vi "GEA3 HEWH Inverter ERD List.vi"(8 "error in (no error)":errorcluster, 11 "Enable Inverter ERD List":bool) -> (0 "error out":errorcluster, 2 "Headers":string[](array[string]), 3 "Read ERD List":T1[](array[typedef]) {"ERD Number" format="%.0x"})   [LabVIEW 2023]
uses:
  type defs/ERD Read Data In.ctl
  type defs/Data Type.ctl
  <vilib>/Utility/error.llb/whitespace.ctl
  <vilib>/Utility/error.llb/Trim Whitespace One-Sided.vi
  library/GEA2_Toolkit.lvlib
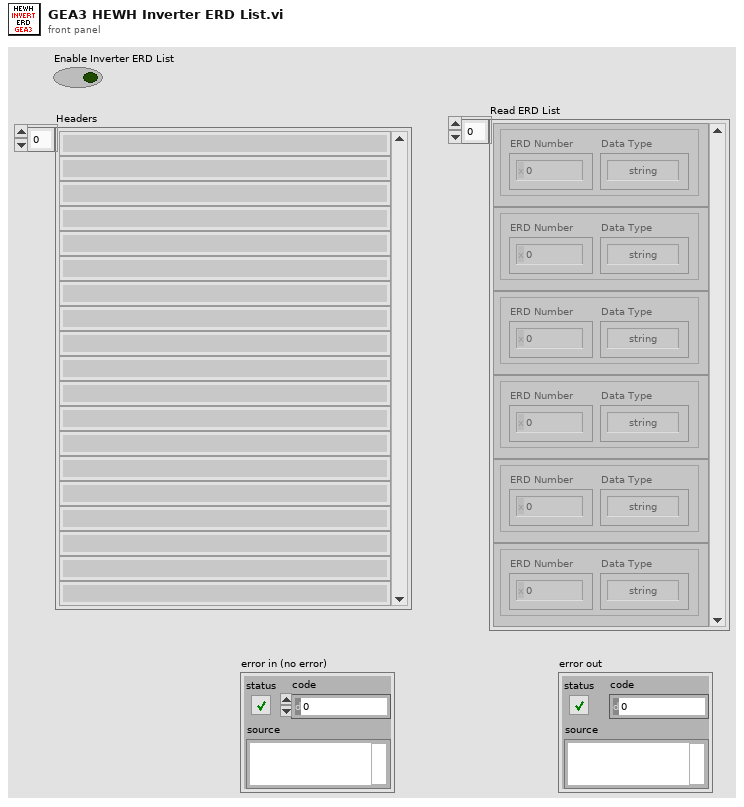
[diagram p1: front panel]
types:
  T1 = typedef "GEA2_Toolkit.lvlib/ERD Read Data In.ctl" = cluster{"ERD Number":u16, "Data Type":T2}
  T2 = typedef "GEA2_Toolkit.lvlib/Data Type.ctl" = enum16{"string", "boolean", "uint8_t", "uint16_t", "uint32_t", "uint64_t", "int8_t", "int16_t", "int32_t", "int64_t"}
  T3 = typedef "whitespace.ctl" = u16
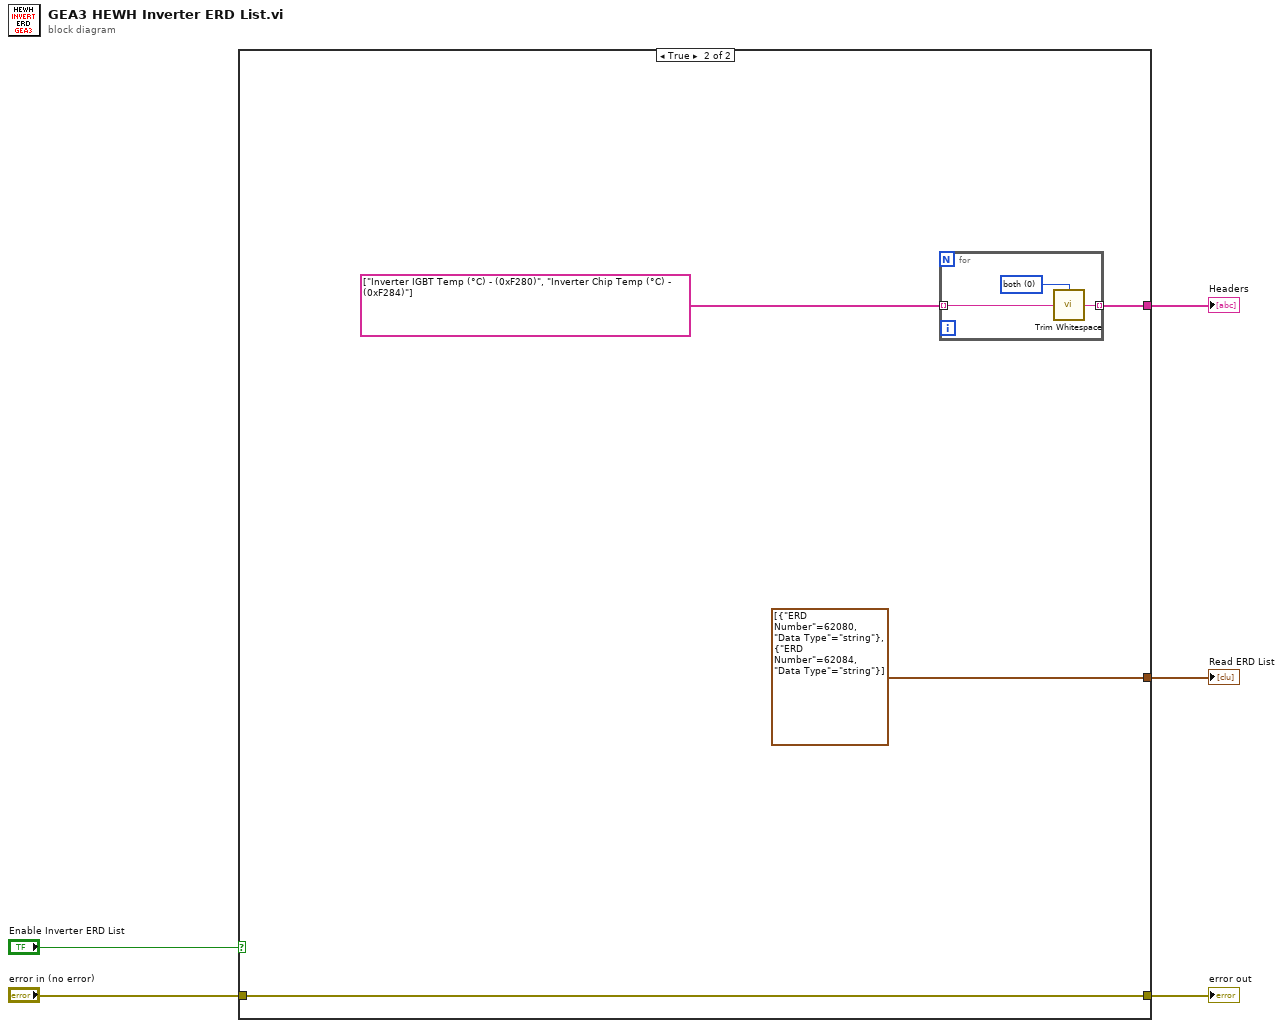
[diagram p0: block diagram]
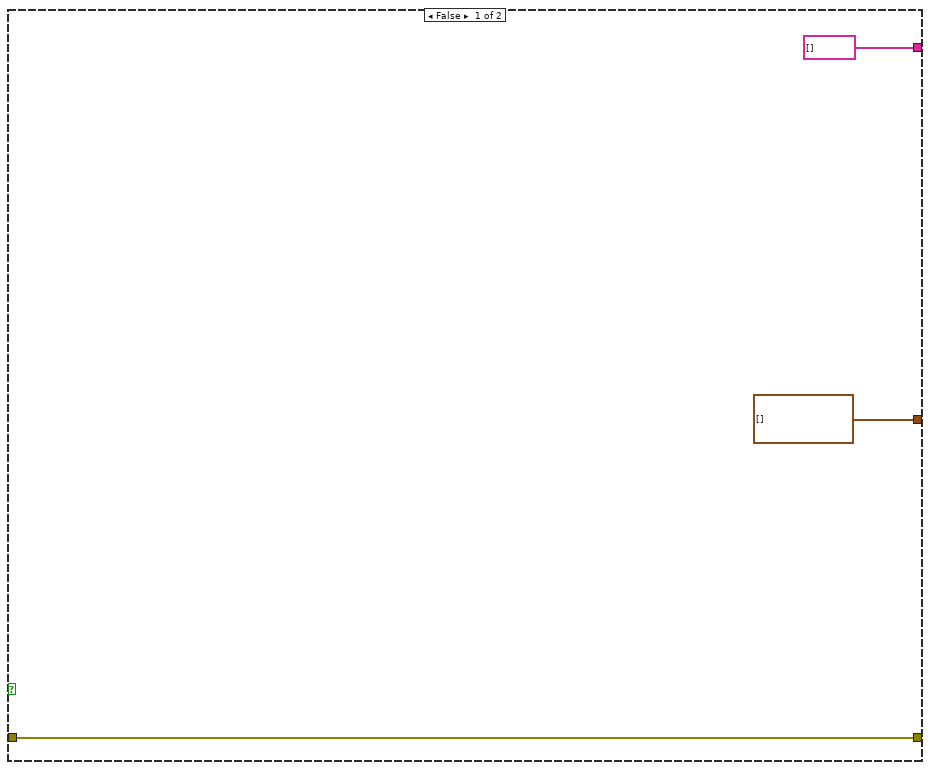
[diagram p2: hidden frame]
diagram:
  n1 = case shown="True" "Enable Inverter ERD List" {
    tunnel: [T1[] [] ("Read ERD List") T1[] [{"ERD Number"=62080, "Data Type"=enum."string"}, {"ERD Number"=62084, "Data Type"=enum."string"}] ("Read ERD List")] -> w5
    tunnel: "error in (no error)" -> [w8 w11]
    tunnel: [w8 w11] -> w3
    tunnel: [string[] [] ("array") w10] -> w1
    frame False {
    }
    frame True {
      n2 = for {
        tunnel: string[] ["Inverter IGBT Temp (°C) - (0xF280)", "Inverter Chip Temp (°C) - (0xF284)"] -> [w14] mode=indexing
        tunnel: [w13] -> w10 mode=indexing
        w15 = T3 0 items=["both", "start of string", "end of string"] ("location (both)")
        n3 = call <vilib>:"Trim Whitespace.vi"("string"=w14, "location (both)"=w15) -> ("trimmed string"=w13:string)
      }
    }
  }
  "Read ERD List" <- w5
  "Headers" <- w1
  "error out" <- w3
